vi "Untitled 1.vi"() -> ()   [LabVIEW 2020]
panel:
  out "String 2":string
  out "String":string
  out "error out":errorcluster
  in  "error in (no error)":errorcluster
  in  "VISA resource name":refnum<visa-resource-name>
  out "Waveform Chart":i32(graph)
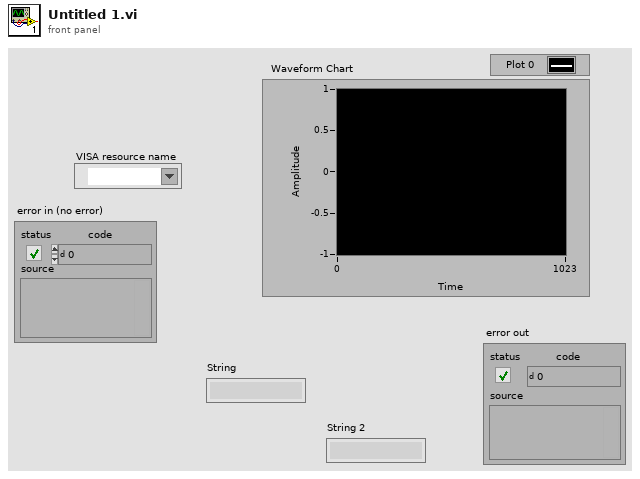
[diagram p1: front panel]
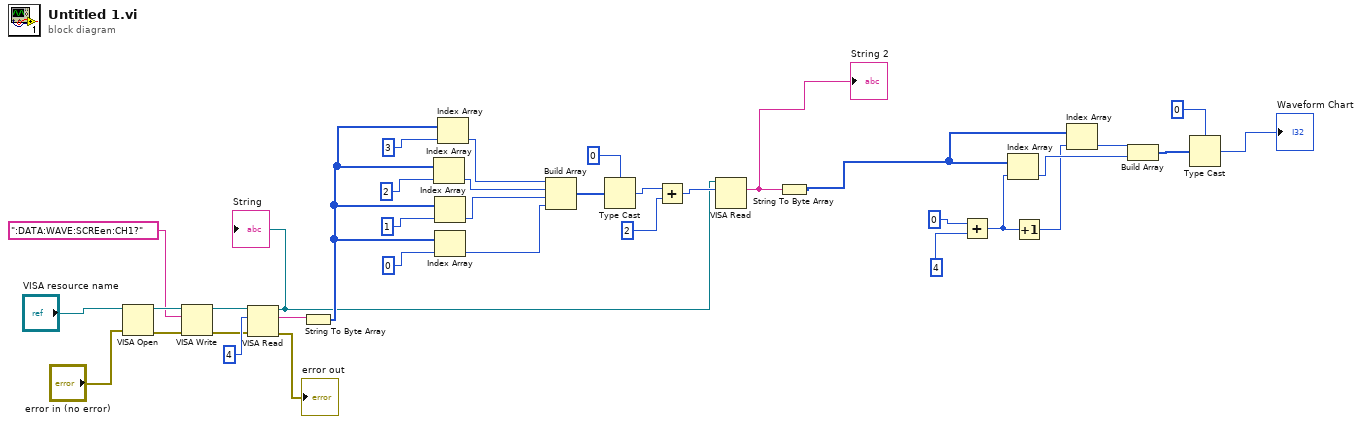
[diagram p0: block diagram]
diagram:
  n1 = VISA Open(error in (no error)="error in (no error)", VISA resource name="VISA resource name") -> (VISA resource name=w4:refnum<visa-resource-name>, error out=w5:errorcluster)  [unwired: 3 in]
  n2 = VISA Write(VISA resource name=w4, write buffer=":DATA:WAVE:SCREen:CH1?", error in (no error)=w5) -> (VISA resource name out=w3:refnum<visa-resource-name>, error out=w2:errorcluster)  [unwired: 1 out]
  n3 = VISA Read(VISA resource name=w3, byte count=4, error in (no error)=w2) -> (VISA resource name out=w9:refnum<visa-resource-name>, read buffer=w36:string, error out=→"error out":errorcluster)  [unwired: 1 out]
  "String" <- w9
  n4 = String To Byte Array(string=w36) -> (unsigned byte array=w24:u8[])
  n5 = Index Array(array=w24, index=2) -> (element=w18:u8)
  n6 = Index Array(array=w24, index=1) -> (element=w17:u8)
  n7 = Index Array(array=w24, index=0) -> (element=w16:u8)
  n8 = Index Array(array=w24, index=3) -> (element=w19:u8)
  n9 = Build Array(w19, w18, w17, w16) -> (w15:u8[])
  n10 = Type Cast(type=0, x=w15) -> (*(type *) &x=w13:i32)
  n11 = Add(x=w13, y=2) -> (x+y=w11:i32)
  n12 = VISA Read(VISA resource name=w9, byte count=w11) -> (read buffer=w6:string)  [unwired: 1 in, 3 out]
  "String 2" <- w6
  n13 = String To Byte Array(string=w6) -> (unsigned byte array=w10:u8[])
  n14 = Add(x=0, y=4) -> (x+y=w29:i32)
  n15 = Index Array(array=w10, index=w29) -> (element=w34:u8)
  n16 = Increment(x=w29) -> (x+1=w30:i32)
  n17 = Index Array(array=w10, index=w30) -> (element=w35:u8)
  n18 = Build Array(w35, w34) -> (w33:u8[])
  n19 = Type Cast(type=0, x=w33) -> (*(type *) &x=→"Waveform Chart":i32)
